vi "ReadMeasurementMetodo.vi"(6 "Measurement Type (0: Frequency)":i32(ring) items=["Frequency", "Mean", "Period", "Pulse Duty", "Peak to Peak", "Cycle RMS", "Minimum", "Maximum", "Rise Time", "Fall Time", "Positive Width", "Negative Width", "Amplitude", "Cycle Mean", "High", "Low", "Negative Duty", "Positive Overshoot", "Negative Overshoot", "Cursor Mean", "Burst Width", "Positive Pulse Count", "Negative Pulse Count", "Rising Edge Count", "Falling Edge Count", "Area", "Cycle Area", "RMS", "Cursor RMS"], 8 "error in (no error)":errorcluster, 9 "Channel (1: Channel 1)":i32(ring)=1 items=["Channel 1"=1, "Channel 2"=2, "Channel 3"=3, "Channel 4"=4], 11 "Keysight in":refnum<class "Edu-1200.lvclass">) -> (0 "error out":errorcluster, 1 "Units":string, 3 "Keysight out":refnum<class "Edu-1200.lvclass">, 4 "Measurement":dbl)   [LabVIEW 2020, in "Edu-1200.lvclass"]
uses:
  Edu-1200.lvclass
  Edu-1200.lvclass/Edu-1200.ctl
  <instrlib>/Agilent 34401/Public/Data/Read (Single Point).vi
  <instrlib>/Agilent 34401/Agilent 34401.lvlib
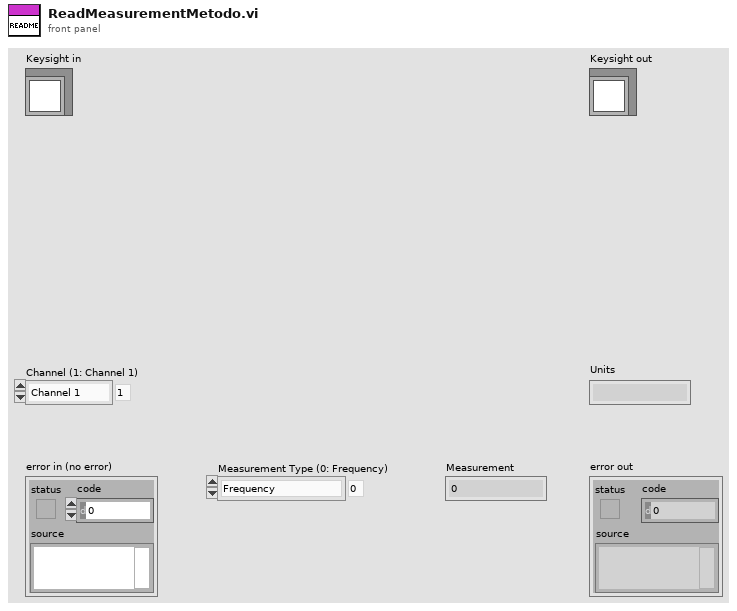
[diagram p1: front panel]
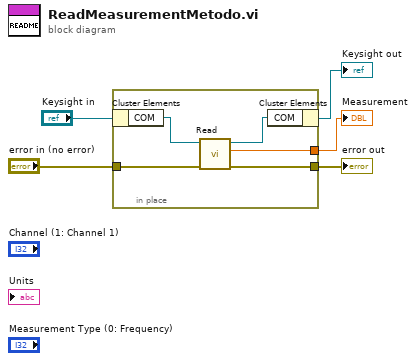
[diagram p0: block diagram]
diagram:
  n1 = in-place {
    in-place-border: [w10] -> w5
    in-place-border: "error in (no error)" -> [w7]
    in-place-border: [w6] -> w3
    n2 = in-place-cluster #1("Keysight in") -> ("COM"=w8:refnum<visa-resource-name>)
    n3 = call-poly <instrlib>:"Read.vi"("error in (no error)"=w7, "VISA resource name"=w8) -> ("error out"=w6:errorcluster, "Measurement"=w10:dbl, "VISA resource name out"=w9:refnum<visa-resource-name>)  [unwired: 7 in]
    n4 = in-place-cluster #1("COM"=w9) -> (→"Keysight out":refnum<class "Edu-1200.lvclass">)
  }
  "error out" <- w3
  "Measurement" <- w5
